vi "Test Google - URL - Build (for stock ticker) - 03.vi"(8 "error in (no error)":errorcluster, 11 "TestCase in":refnum<class "TestCase.lvclass">) -> (0 "error out":errorcluster, 3 "TestCase out":refnum<class "TestCase.lvclass">)   [LabVIEW 2011, in "test.lvclass"]
uses:
  test.lvclass
  <vilib>/addons/_JKI Toolkits/VI Tester/TestCase.llb/TestCase.lvclass
  src/Stock Data Control.ctl
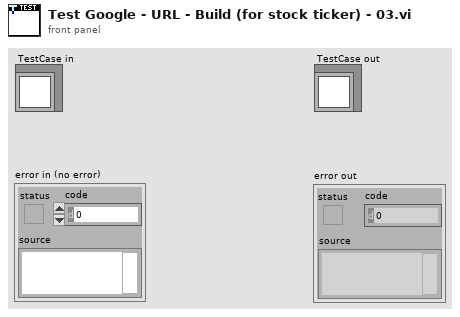
[diagram p1: front panel]
types:
  T1 = typedef "Stock Data Control.ctl" = cluster{"Symbol":string, "Name":string, "Price":string, "Change":string, "Change %":string, "Volume":string}
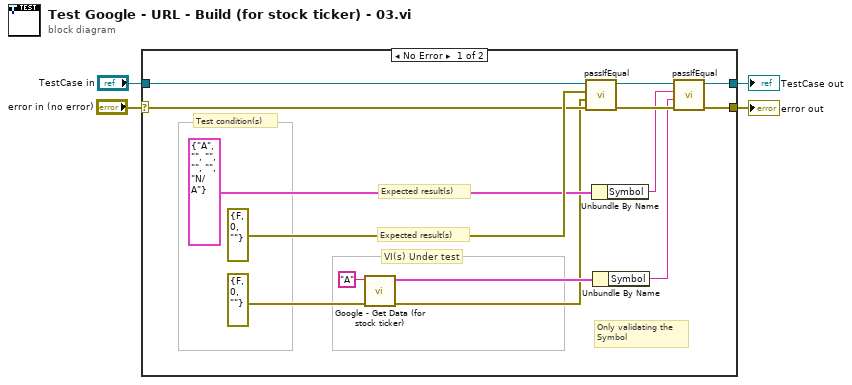
[diagram p0: block diagram]
diagram:
  n1 = case shown="No Error" "error in (no error)" {
    selector: "error in (no error)" -> [w14 w19]
    tunnel: "TestCase in" -> [w15 w20]
    tunnel: [w12 w20] -> w3
    tunnel: [w13 w19] -> w2
    frame No Error {
      # "Only validating the\nSymbol"
      # "Expected result(s)"
      # "Expected result(s)"
      # "Test condition(s)"
      # "VI(s) Under test"
      n2 = call "Google - Get Data (for stock ticker).vi"("Symbol"="A", "error in"=errorcluster {"status"=FALSE, "code"=0, "source"=""} ("error in (no error)")) -> ("Stock Data"=w6:T1, "error out"=w5:errorcluster)  [unwired: 6 in]
      n3 = call-dynamic "passIfEqual.vi"("error in (no error)"=w14, "y"=w5, "x"=errorcluster {"status"=FALSE, "code"=0, "source"=""} ("error in (no error)"), "TestCase in"=w15) -> ("error out"=w10:errorcluster, "TestCase out"=w11:refnum<class "TestCase.lvclass">)  [unwired: 6 in]
      n4 = Unbundle By Name(T1 {"Symbol"="A", "Name"="", "Price"="", "Change"="", "Change %"="", "Volume"="N/A"} ("Stock Data")) -> ("Symbol"=w8:string)
      n5 = Unbundle By Name(w6) -> ("Symbol"=w7:string)
      n6 = call-dynamic "passIfEqual.vi"("error in (no error)"=w10, "y"=w7, "x"=w8, "TestCase in"=w11) -> ("error out"=w13:errorcluster, "TestCase out"=w12:refnum<class "TestCase.lvclass">)  [unwired: 6 in]
    }
    frame Error {
    }
  }
  "TestCase out" <- w3
  "error out" <- w2
